vi "Simulation Data_Global.vi"() -> ()   [LabVIEW 2025, in "Simulated Evaporative Cooler.lvclass"]
doc: "This global VI defines all the values used in the simulation of the evaporative cooler. The panel of this global may be used during the simulation to monitor and/or adjust parameters."
uses:
  Simulated Evaporative Cooler.lvclass
panel:
  in  "Outdoor Temperature":dbl=110.0
  out "Water Level":dbl
  out "Water Valve State":bool
  out "Indoor Temperature":dbl
  out "Fan A State":bool
  out "Fan B State":bool
  in  "Fan B Fault":bool
  in  "Fan A Fault":bool
  # "This panel may be used during the simulation to monitor and/or adjust parameters."
  # "Simulation Inputs"
  # "Simulation Outputs"
  # "Adjust these to change condition of the system."
  # "Observe these to see the response of the system."
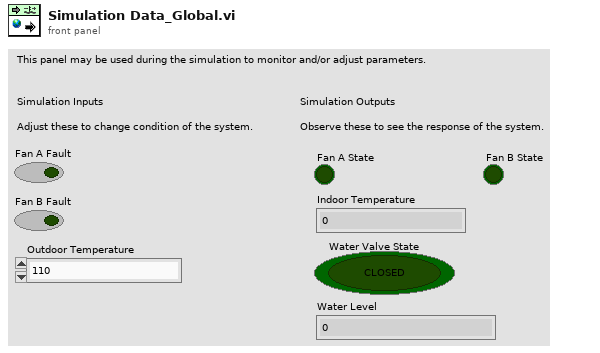
[diagram p1: front panel]
diagram:
